vi "Read_IntakeCommand.vi"(8 "error in (no error)":errorcluster, 11 "IntakeData in":refnum<class "IntakeData.lvclass">) -> (0 "error out":errorcluster, 2 "Intake Command":T1, 3 "IntakeData out":refnum<class "IntakeData.lvclass">)   [LabVIEW 2017, in "IntakeData.lvclass"]
uses:
  IntakeData.lvclass
  Team-code/IntakeCommand.ctl
  IntakeData.lvclass/IntakeData.ctl
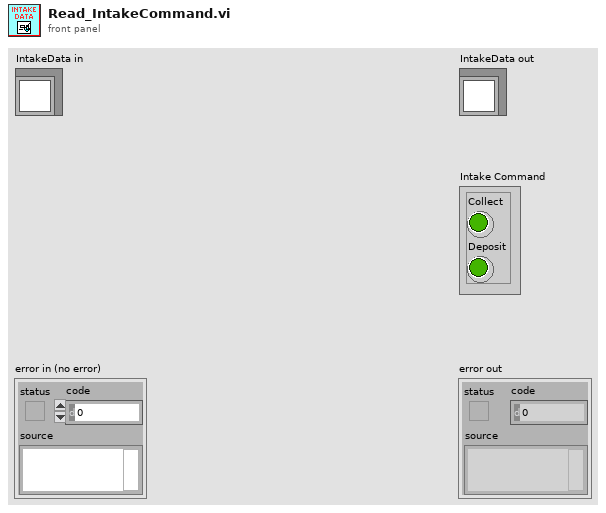
[diagram p1: front panel]
types:
  T1 = typedef "IntakeData.lvclass/IntakeCommand.ctl" = cluster{"Collect":bool, "Deposit":bool}
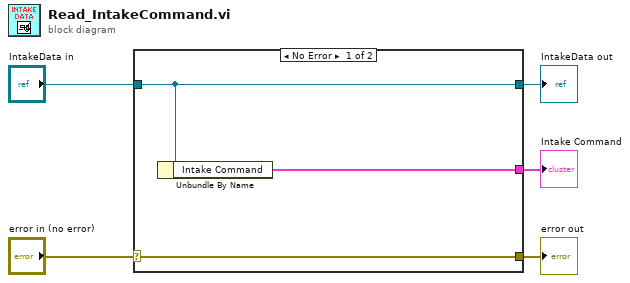
[diagram p0: block diagram]
diagram:
  n1 = case shown="No Error" "error in (no error)" {
    selector: "error in (no error)" -> [w8 w9]
    tunnel: [w8 w9] -> w4
    tunnel: [w7 w10] -> w2
    tunnel: "IntakeData in" -> [w7 w10]
    tunnel: [w6 _] -> w1
    frame No Error {
      n2 = Unbundle By Name(w7) -> ("Intake Command"=w6:T1)
    }
    frame Error {
    }
  }
  "error out" <- w4
  "IntakeData out" <- w2
  "Intake Command" <- w1
